vi "4.vi"   [LabVIEW 2018]
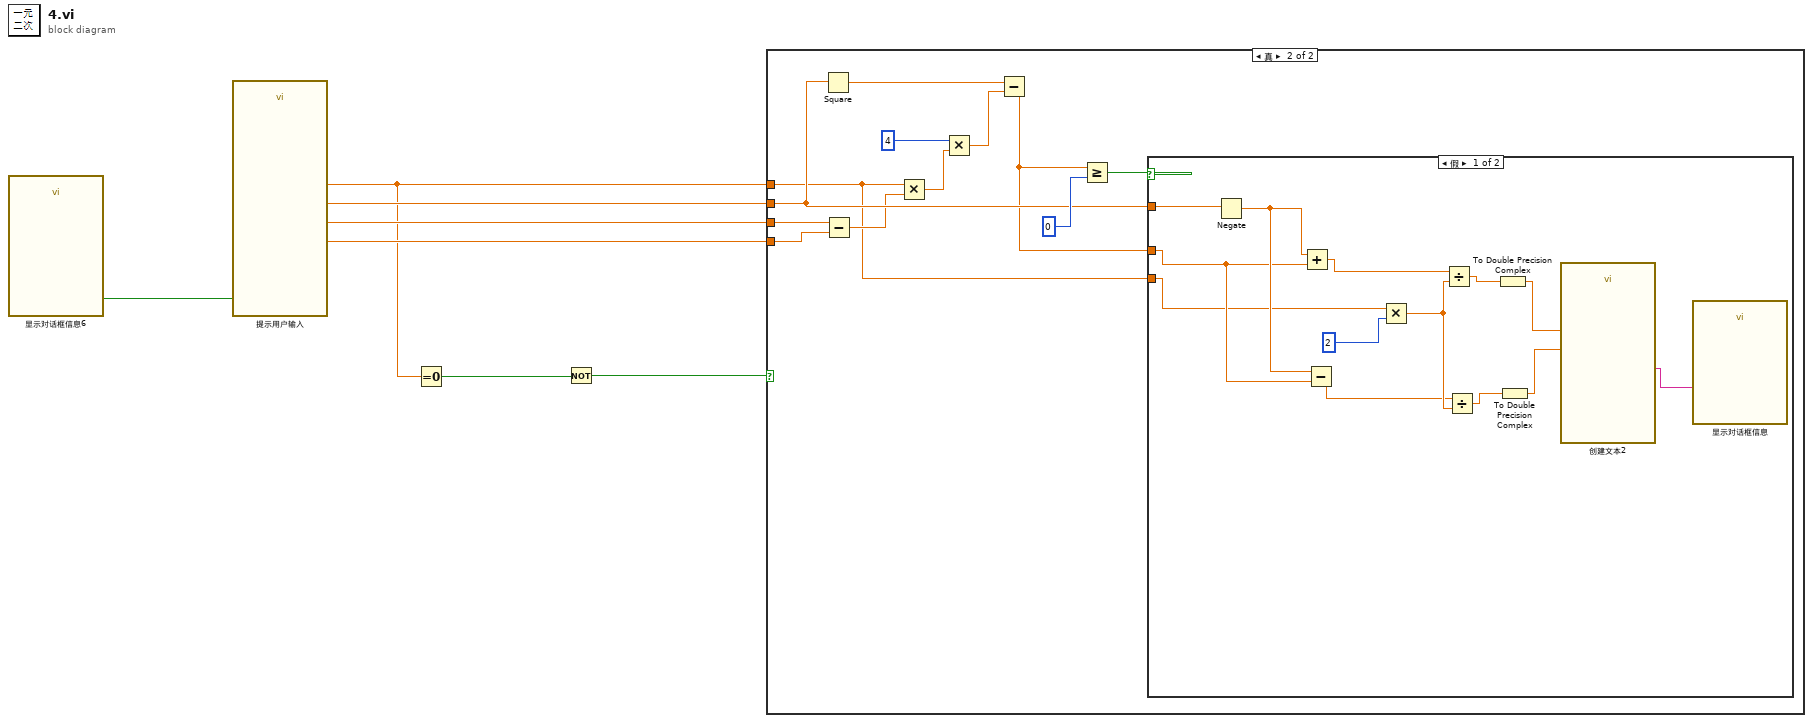
[diagram p0: block diagram]
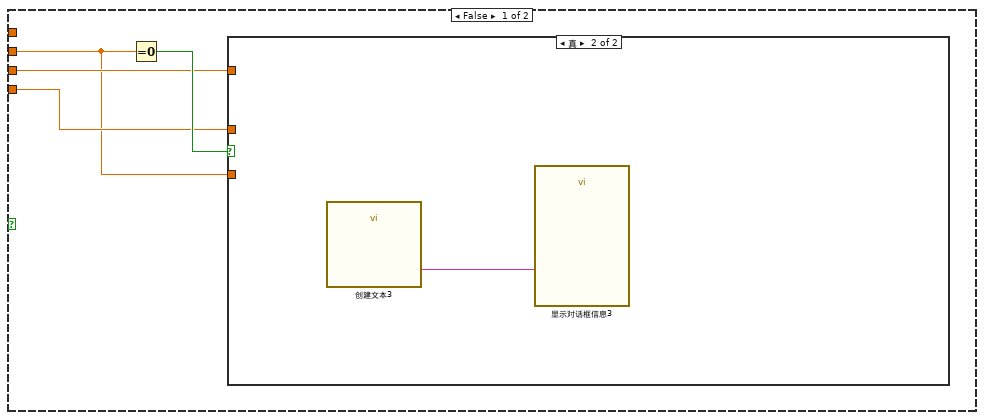
[diagram p2: hidden frame]
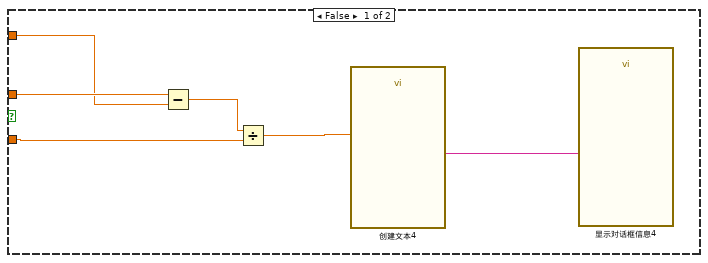
[diagram p3: hidden frame]
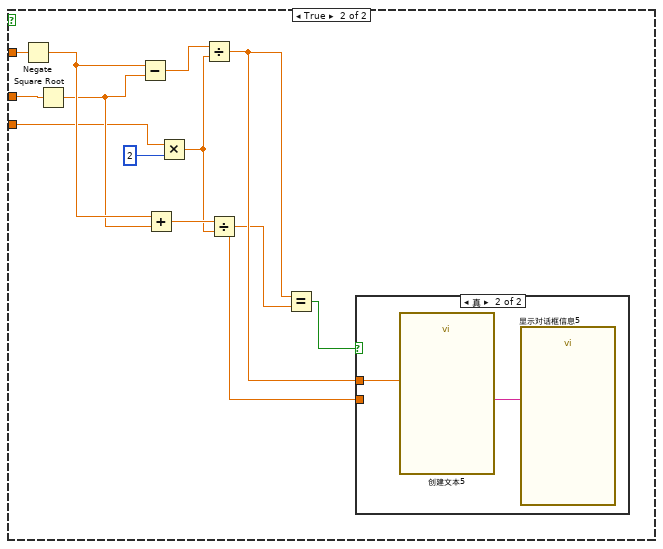
[diagram p4: hidden frame]
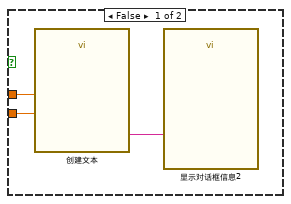
[diagram p5: hidden frame]
diagram:
  n1 = call "显示对话框信息6"() -> ("确定"=w1:bool)  [unwired: 10 in, 1 out]
  n2 = call "提示用户输入"("Enable"=w1) -> ("D"=w5:dbl, "C"=w6:dbl, "B"=w7:dbl, "A"=w4:dbl)  [unwired: 13 in, 2 out]
  n3 = Equal To 0?(x=w4) -> (x = 0?=w3:bool)
  n4 = Not(x=w3) -> (.not. x?=w2:bool)
  n5 = case shown="真" w2 {
    tunnel: w7 -> [w8 w25]
    tunnel: w6 -> [w9 w22]
    tunnel: w5 -> [w10 w21]
    tunnel: w4 -> [_ w19]
    frame False {
      n6 = Equal To 0?(x=w8) -> (x = 0?=w11:bool)
      n7 = case shown="真" w11 {
        tunnel: w10 -> [w17 _]
        tunnel: w9 -> [w16 _]
        tunnel: w8 -> [w14 _]
        frame False {
          n8 = Subtract(x=w17, y=w16) -> (x-y=w15:dbl)
          n9 = Divide(x=w15, y=w14) -> (x/y=w13:dbl)
          n10 = call "创建文本4"("a"=w13) -> ("Result"=w12:string)  [unwired: 13 in, 1 out]
          n11 = call "显示对话框信息4"("Message"=w12) -> ()  [unwired: 9 in, 2 out]
        }
        frame True {
          n12 = call "创建文本3"() -> ("Result"=w18:string)  [unwired: 14 in, 1 out]
          n13 = call "显示对话框信息3"("Message"=w18) -> ()  [unwired: 9 in, 2 out]
        }
      }
    }
    frame True {
      n14 = Square(x=w25) -> (x^2=w29:dbl)
      n15 = Subtract(x=w22, y=w21) -> (x-y=w20:dbl)
      n16 = Multiply(x=w19, y=w20) -> (x*y=w23:dbl)
      n17 = Multiply(x=4, y=w23) -> (x*y=w28:dbl)
      n18 = Subtract(x=w29, y=w28) -> (x-y=w24:dbl)
      n19 = Greater Or Equal?(x=w24, y=0) -> (x >= y?=w26:bool)
      n20 = case shown="假" w26 {
        tunnel: w25 -> [w43 w55]
        tunnel: w24 -> [w41 w54]
        tunnel: w19 -> [w39 w51]
        frame False {
          n21 = Negate(x=w43) -> (-x=w42:dbl)
          n22 = Add(x=w42, y=w41) -> (x+y=w38:dbl)
          n23 = Subtract(x=w42, y=w41) -> (x-y=w36:dbl)
          n24 = Multiply(x=w39, y=2) -> (x*y=w37:dbl)
          n25 = Divide(x=w38, y=w37) -> (x/y=w34:dbl)
          n26 = Divide(x=w36, y=w37) -> (x/y=w32:dbl)
          n27 = To Double Precision Complex(1:w34) -> (0:w33:cdb)
          n28 = To Double Precision Complex(1:w32) -> (0:w31:cdb)
          n29 = call "创建文本2"("a"=w33, "b"=w31) -> ("Result"=w35:string)  [unwired: 12 in, 1 out]
          n30 = call "显示对话框信息"("Message"=w35) -> ()  [unwired: 9 in, 2 out]
        }
        frame True {
          n31 = Negate(x=w55) -> (-x=w53:dbl)
          n32 = Square Root(x=w54) -> (sqrt(x)=w52:dbl)
          n33 = Subtract(x=w53, y=w52) -> (x-y=w49:dbl)
          n34 = Add(x=w53, y=w52) -> (x+y=w48:dbl)
          n35 = Multiply(x=w51, y=2) -> (x*y=w47:dbl)
          n36 = Divide(x=w49, y=w47) -> (x/y=w45:dbl)
          n37 = Divide(x=w48, y=w47) -> (x/y=w44:dbl)
          n38 = Equal?(x=w45, y=w44) -> (x = y?=w46:bool)
          n39 = case shown="真" w46 {
            tunnel: w45 -> [w58 w59]
            tunnel: w44 -> [w57 _]
            frame False {
              n40 = call "创建文本"("A"=w58, "B"=w57) -> ("Result"=w56:string)  [unwired: 12 in, 1 out]
              n41 = call "显示对话框信息2"("Message"=w56) -> ()  [unwired: 9 in, 2 out]
            }
            frame True {
              n42 = call "创建文本5"("a"=w59) -> ("Result"=w60:string)  [unwired: 13 in, 1 out]
              n43 = call "显示对话框信息5"("Message"=w60) -> ()  [unwired: 9 in, 2 out]
            }
          }
        }
      }
    }
  }
